vi "MovePiece.vi"(7 "Old piece":i32[][](array[numeric]), 8 "Down":bool, 9 "Right":bool, 10 "Left":bool, 11 "Up":bool) -> (3 "New piece":i32[][](array[numeric]))   [LabVIEW 2014]
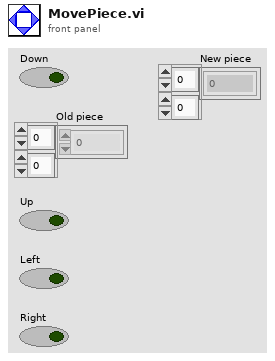
[diagram p1: front panel]
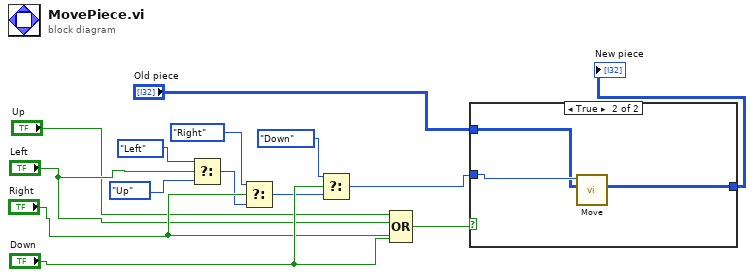
[diagram p0: block diagram]
diagram:
  n1 = Select(t=enum16{"Up", "Left", "Right", "Down"}."Left", s="Left", f=enum16{"Up", "Left", "Right", "Down"}."Up") -> (s? t:f=w3:enum16{"Up", "Left", "Right", "Down"})
  n2 = Select(t=enum16{"Up", "Left", "Right", "Down"}."Right", s="Right", f=w3) -> (s? t:f=w6:enum16{"Up", "Left", "Right", "Down"})
  n3 = Select(t=enum16{"Up", "Left", "Right", "Down"}."Down", s="Down", f=w6) -> (s? t:f=w8:enum16{"Up", "Left", "Right", "Down"})
  n4 = Compound Arithmetic op=OR("Up", "Left", "Right", "Down") -> (w5:bool)
  n5 = case shown="True" w5 {
    tunnel: w8 -> [_ w18]
    tunnel: "Old piece" -> [w15 w17]
    tunnel: [w15 w16] -> w14
    frame False {
    }
    frame True {
      n6 = call "Move.vi"("Piece"=w17, "Enum"=w18) -> ("New piece"=w16:i32[][])  [unwired: 9 in]
    }
  }
  "New piece" <- w14
